vi "enqueue test results.vi"(8 "error in":errorcluster, 10 "test results":T1, 11 "queue in":refnum<queue>) -> (0 "error out":errorcluster, 3 "queue out 2":refnum<queue>)   [LabVIEW 2020]
uses:
  Inverter/controls/INV_test results.ctl
  Inverter/controls/Inverter_step_type.ctl
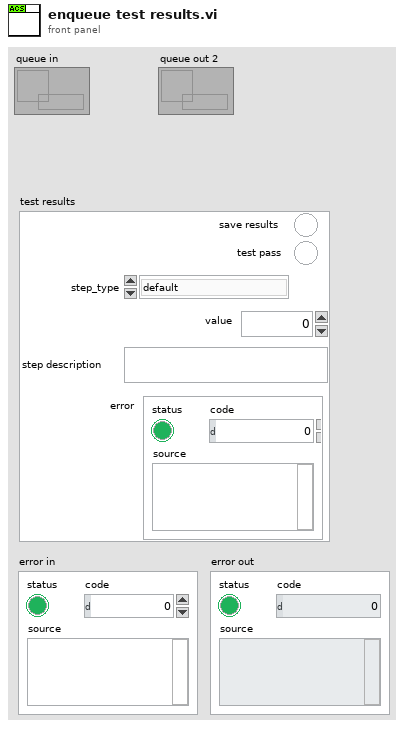
[diagram p1: front panel]
types:
  T1 = typedef "INV_test results.ctl" = cluster{"test pass":bool, "step_type":T2, "value":dbl, "step description":string, "error":errorcluster, "save results":bool}
  T2 = typedef "Inverter_step_type.ctl" = enum16{"default", "prompt", "sequence#", "12V_1_power supply on_off", "12V_2_power supply on_off", "write_PLC", "read_PLC", "wait (sec)", "record_pass_fail"}
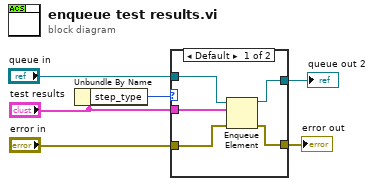
[diagram p0: block diagram]
diagram:
  n1 = Unbundle By Name("test results") -> ("step_type"=w1:T2)
  n2 = case shown="Default" w1 {
    tunnel: "error in" -> [w11 w12]
    tunnel: [w10 w12] -> w5
    tunnel: "queue in" -> [w9 w13]
    tunnel: [w8 w13] -> w3
    tunnel: "test results" -> [w7 _]
    frame Default {
      n3 = Enqueue Element(queue=w9, element=w7, error in (no error)=w11) -> (queue out=w8:refnum<queue>, error out=w10:errorcluster)  [unwired: 1 in, 1 out]
    }
    frame "default" {
    }
  }
  "error out" <- w5
  "queue out 2" <- w3
